vi "OpenImageFromFile.vi"(8 "error in (no error)":errorcluster, 11 "File Path":path) -> (0 "error out":errorcluster, 3 "Image":T1(plugin-control))   [LabVIEW 2019]
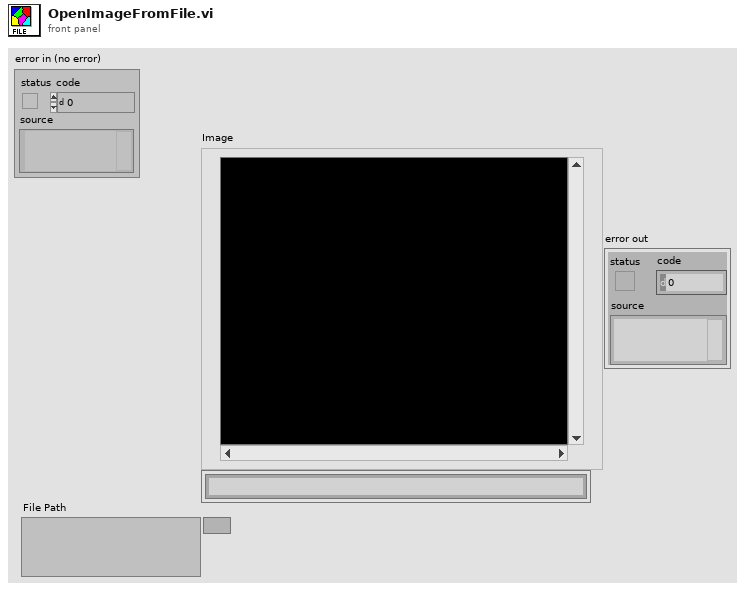
[diagram p1: front panel]
types:
  T1 = typedef "IMAQ Image.ctl" = refnum<image>
  T2 = typedef "Image Type" = u32
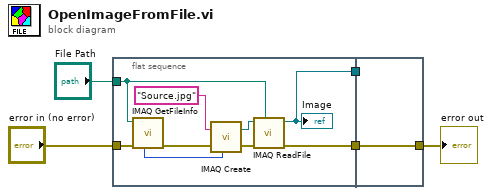
[diagram p0: block diagram]
diagram:
  n1 = flat-sequence {
    tunnel: [w10] -> w5
    tunnel: [w8] -> w4
    tunnel: "File Path" -> [w9]
    tunnel: "error in (no error)" -> [w6]
    tunnel: w5 -> [w15]
    tunnel: w4 -> [_]
    tunnel: [w15] -> w3
    frame #0 {
      n2 = call "IMAQ GetFileInfo"("error in (no error)"=w6, "File Path"=w9) -> ("error out"=w12:errorcluster, "Image Type"=w13:T2)  [unwired: 8 out]
      n3 = call "IMAQ Create"("Image Name"="Source.jpg", "Image Type"=w13, "error in (no error)"=w12) -> ("New Image"=w14:T1, "error out"=w7:errorcluster)  [unwired: 1 in, 1 out]
      n4 = call "IMAQ ReadFile"("File Path"=w9, "error in (no error)"=w7, "Image"=w14) -> ("error out"=w10:errorcluster, "Image Out"=w8:T1)  [unwired: 2 in, 5 out]
      "Image" <- w8
    }
    frame #1 {
    }
  }
  "error out" <- w3
